vi "Load Controller Type from Enum.vi"(8 "error in (no error)":errorcluster, 11 "Controller Type":T1) -> (0 "error out":errorcluster, 3 "controller out":refnum<class "Generic Plugin.lvclass">)   [LabVIEW 2020, in "Generic Plugin.lvclass"]
uses:
  Generic Plugin.lvclass
  File IO/File IO.lvlib
  Controller Type.ctl
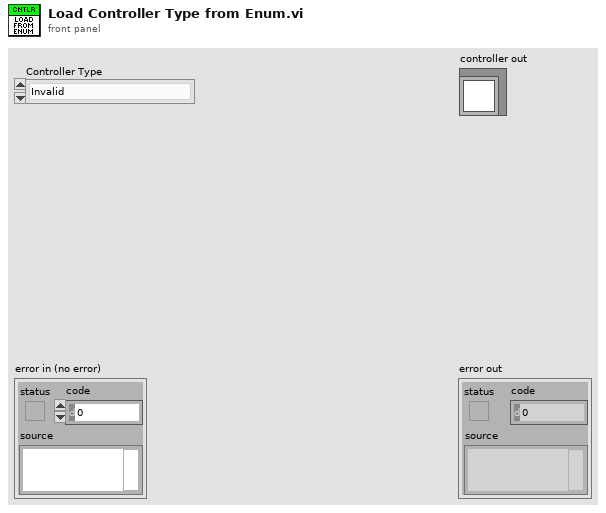
[diagram p1: front panel]
types:
  T1 = typedef "Generic Plugin.lvclass/Controller Type.ctl" = enum16{"Invalid", "Temperature Controller", "Pump Controller", "Generic Optimizer", "LC Parser"}
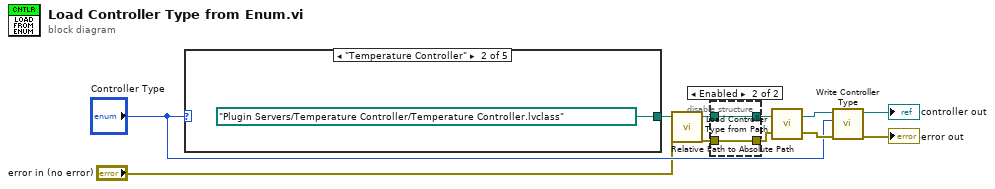
[diagram p0: block diagram]
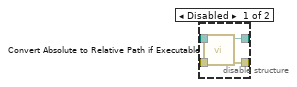
[diagram p2: hidden frame]
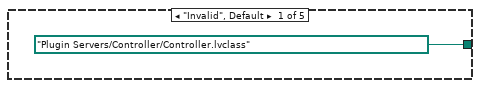
[diagram p3: hidden frame]
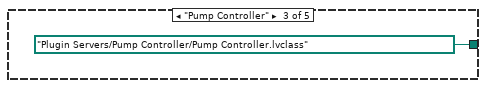
[diagram p4: hidden frame]
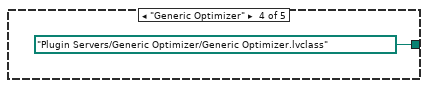
[diagram p5: hidden frame]
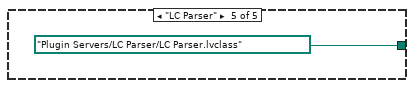
[diagram p6: hidden frame]
diagram:
  n1 = case shown="\"Temperature Controller\"" "Controller Type" {
    tunnel: [path "Plugin Servers/Controller/Controller.lvclass" path "Plugin Servers/Temperature Controller/Temperature Controller.lvclass" path "Plugin Servers/Pump Controller/Pump Controller.lvclass" path "Plugin Servers/Generic Optimizer/Generic Optimizer.lvclass" path "Plugin Servers/LC Parser/LC Parser.lvclass"] -> w10
    frame "Invalid", Default {
    }
    frame "Temperature Controller" {
    }
    frame "Pump Controller" {
    }
    frame "Generic Optimizer" {
    }
    frame "LC Parser" {
    }
  }
  n2 = call "Relative Path to Absolute Path.vi"("Relative Path"=w10) -> ("Absolute Path"=w4:path)  [unwired: 4 in]
  n3 = disable-structure shown="Enabled" {
    disable-tunnel: w4 -> [w19 w21]
    disable-tunnel: [w18 w21] -> w3
    disable-tunnel: "error in (no error)" -> [w17 w20]
    disable-tunnel: [w16 w20] -> w1
    frame Disabled {
      n4 = call "Convert Absolute to Relative Path if Executable.vi"("error in (no error)"=w17, "Absolute Path"=w19) -> ("error out"=w16:errorcluster, "Result Path"=w18:path)  [unwired: 7 in, 1 out]
    }
    frame Enabled {
    }
  }
  n5 = call "Load Controller Type from Path.vi"("error in (no error)"=w1, "Absolute Path"=w3) -> ("error out"=w7:errorcluster, "Controller out"=w9:refnum<class "Generic Plugin.lvclass">)
  n6 = call "Write Controller Type.vi"("error in (no error)"=w7, "Controller Type"="Controller Type", "Generic Controller in"=w9) -> ("error out"=→"error out":errorcluster, "Generic Controller out"=→"controller out":refnum<class "Generic Plugin.lvclass">)  [unwired: 7 in]
